vi "Manage Accounts.vi"(7 "Action":T1(ring), 8 "error in (no error)":errorcluster, 10 "Set Value":string, 11 "PIN":string) -> (0 "error out":errorcluster, 2 "Get Value":string)   [LabVIEW 2012]
doc: "This VI manages the account records and the file that stores them on disk. It provides encapsulation for the record data so that the file structure or data set can be changed, and this functions callers will not have to be updated to accommodate those changes."
uses:
  Controls/Account Info.ctl
  <vilib>/Utility/file.llb/Read From Spreadsheet File (string).vi
  <vilib>/Utility/file.llb/Write To Spreadsheet File (string).vi
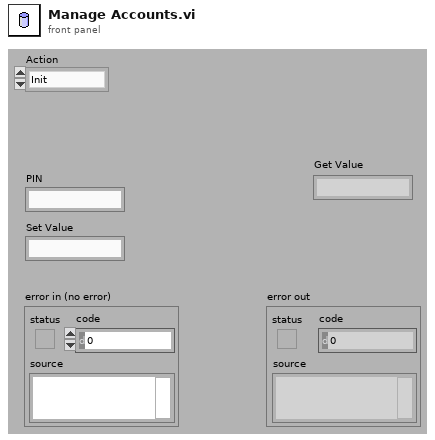
[diagram p1: front panel]
types:
  T1 = enum16{"Init", "Get Balance", "Update Balance", "Find Name"}
  T2 = typedef "Account Info.ctl" = cluster{"PIN":string, "First":string, "Last":string, "Amount":string}
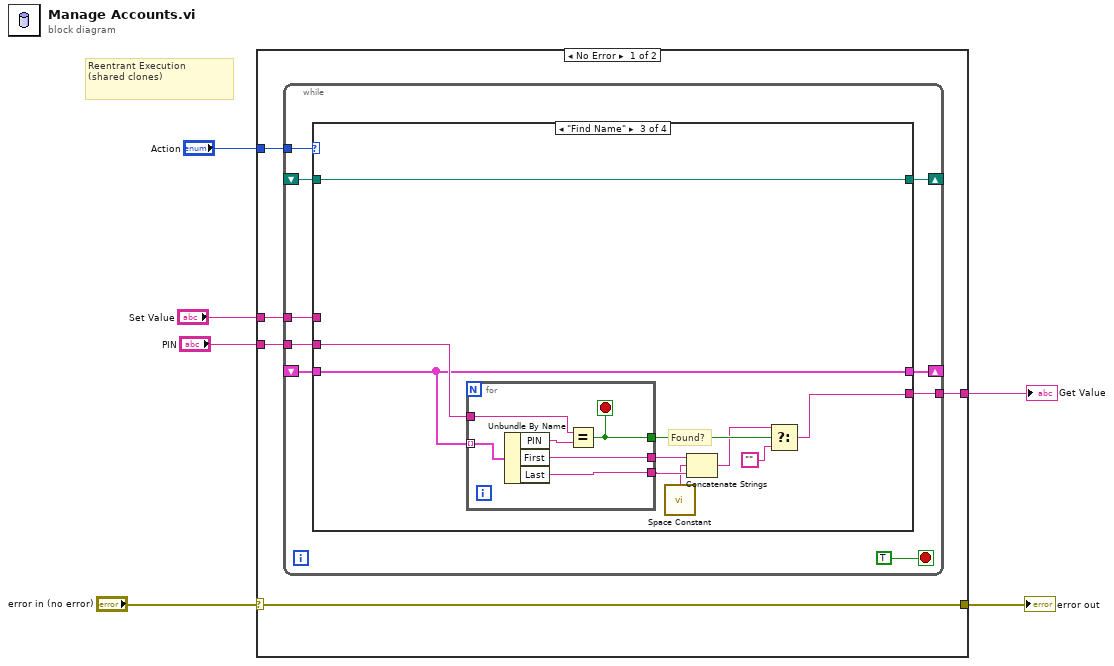
[diagram p0: block diagram]
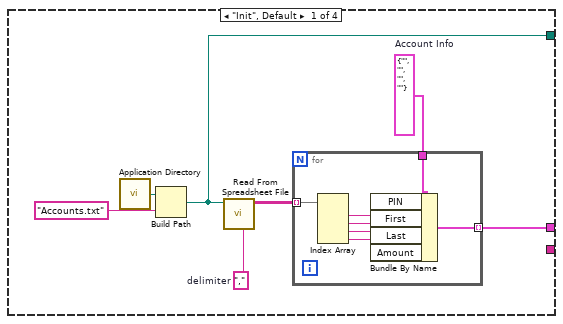
[diagram p2: hidden frame]
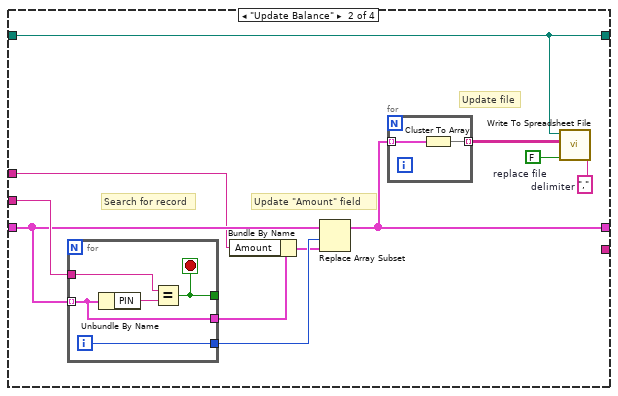
[diagram p3: hidden frame]
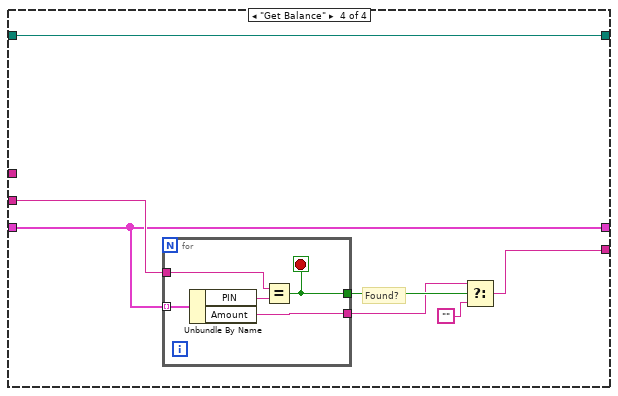
[diagram p4: hidden frame]
diagram:
  # "Reentrant Execution\n(shared clones)"
  n1 = case shown="No Error" "error in (no error)" {
    selector: "error in (no error)" -> [w11 w81]
    tunnel: [w11 w81] -> w5
    tunnel: "Action" -> [w10 _]
    tunnel: "PIN" -> [w9 _]
    tunnel: [w8 _] -> w2
    tunnel: "Set Value" -> [w7 _]
    frame No Error {
      n2 = while {
        shift-right: [w19] -> _
        shift-left: _ -> [w18]
        tunnel: w10 -> [w17]
        tunnel: w9 -> [w16]
        tunnel: [w15] -> w8
        tunnel: w7 -> [w14]
        shift-right: [w13] -> _
        shift-left: _ -> [w12]
        stop <- TRUE stop-if-true
        n3 = case shown="\"Find Name\"" w17 {
          tunnel: [w23 w38 w54 w71] -> w19
          tunnel: w18 -> [_ w44 w54 w71]
          tunnel: w16 -> [_ w45 w62 w75]
          tunnel: [_ _ w55 w72] -> w15
          tunnel: w14 -> [_ w40 _ _]
          tunnel: [w21 w39 w53 w69] -> w13
          tunnel: w12 -> [_ w39 w53 w69]
          frame "Init", Default {
            w22 = T2 {"PIN"="", "First"="", "Last"="", "Amount"=""}  # Account Info
            w27 = ","  # delimiter
            n4 = call <vilib>:"Application Directory.vi"() -> ("Application Directory"=w24:path)
            n5 = Build Path(base path=w24, name or relative path="Accounts.txt") -> (appended path=w21:path)
            n6 = call-poly <vilib>:"Read From Spreadsheet File.vi"("delimiter (\\t)"=w27, "file path (dialog if empty)"=w21) -> ("all rows"=w25:string[][])  [unwired: 5 in, 4 out]
            n7 = for {
              tunnel: w25 -> [w34] mode=indexing
              tunnel: [w29] -> w23 mode=indexing
              tunnel: w22 -> [w28]
              n8 = Index Array(array=w34) -> (element #1=w33:string, element #2=w32:string, element #3=w31:string, element #4=w30:string)  [unwired: 4 in]
              n9 = Bundle By Name(cluster=w28, "PIN"=w33, "First"=w32, "Last"=w31, "Amount"=w30) -> (w29:T2)
            }
          }
          frame "Update Balance" {
            w35 = ","  # delimiter
            w36 = FALSE  # replace file
            # "Update file"
            # "Update \"Amount\" field"
            # "Search for record"
            n10 = for {
              tunnel: w44 -> [w48] mode=indexing
              tunnel: w45 -> [w51]
              tunnel: [w50] -> _
              tunnel: [w49] -> w43
              tunnel: [w48] -> w42
              i -> [w49]
              stop <- w50 stop-if-true
              n11 = Unbundle By Name(w48) -> ("PIN"=w52:string)
              n12 = Equal?(x=w51, y=w52) -> (x = y?=w50:bool)
            }
            n13 = Bundle By Name(cluster=w42, "Amount"=w40) -> (w41:T2)
            n14 = Replace Array Subset(array=w44, new element=w41, index=w43) -> (w38:T2[])
            n15 = for {
              tunnel: w38 -> [w47] mode=indexing
              tunnel: [w46] -> w37 mode=indexing
              n16 = Cluster To Array(cluster=w47) -> (array=w46:string[])
            }
            n17 = call-poly <vilib>:"Write To Spreadsheet File.vi"("delimiter (\\t)"=w35, "append to file? (new file:F)"=w36, "2D data"=w37, "file path (dialog if empty)"=w39) -> ()  [unwired: 4 in, 1 out]
          }
          frame "Find Name" {
            # "Found?"
            n18 = for {
              tunnel: w54 -> [w68] mode=indexing
              tunnel: w62 -> [w66]
              tunnel: [w65] -> w58
              tunnel: [w64] -> w61
              tunnel: [w63] -> w60
              stop <- w65 stop-if-true
              n19 = Unbundle By Name(w68) -> ("PIN"=w67:string, "First"=w64:string, "Last"=w63:string)
              n20 = Equal?(x=w66, y=w67) -> (x = y?=w65:bool)
            }
            n21 = call <vilib>:"Space Constant.vi"() -> ("String"=w59:string)
            n22 = Concatenate Strings(w61, w59, w60) -> (w57:string)
            n23 = Select(t=w57, s=w58, f="") -> (s? t:f=w55:string)
          }
          frame "Get Balance" {
            # "Found?"
            n24 = for {
              tunnel: w71 -> [w80] mode=indexing
              tunnel: w75 -> [w78]
              tunnel: [w77] -> w74
              tunnel: [w76] -> w70
              stop <- w77 stop-if-true
              n25 = Unbundle By Name(w80) -> ("PIN"=w79:string, "Amount"=w76:string)
              n26 = Equal?(x=w78, y=w79) -> (x = y?=w77:bool)
            }
            n27 = Select(t=w70, s=w74, f="") -> (s? t:f=w72:string)
          }
        }
      }
    }
    frame Error {
    }
  }
  "error out" <- w5
  "Get Value" <- w2
